vi "TLCCS Get Device Status.vi"(8 "error in (no error)":errorcluster {"code" format="%.0x"}, 11 "instrument handle":refnum<visa-resource-name>) -> (0 "error out":errorcluster {"code" format="%.0x"}, 2 "Device Status":i32, 3 "instrument handle out":refnum<visa-resource-name>)   [LabVIEW 2020]
doc: "This VI retrieves the status of the CCS. You can use this VI to detect if an external trigger has already occurred.\n\nNote:\nThe values anove are defined in the drivers header file."
uses:
  tlccs_32.dll
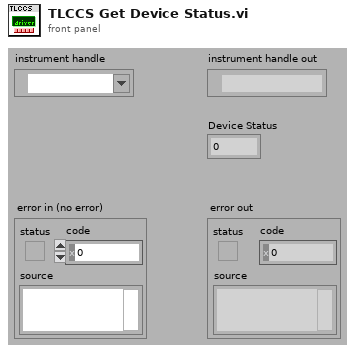
[diagram p1: front panel]
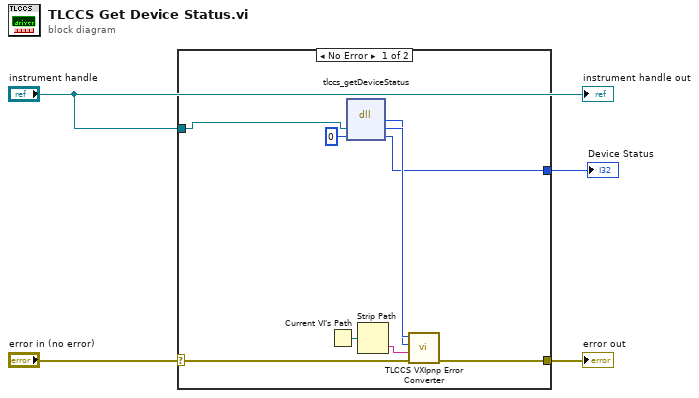
[diagram p0: block diagram]
diagram:
  n1 = case shown="No Error" "error in (no error)" {
    selector: "error in (no error)" -> [w8 w14]
    tunnel: [w7 w14] -> w4
    tunnel: "instrument handle" -> [w12 _]
    tunnel: [w5 _] -> w1
    frame No Error {
      n2 = Current VI's Path() -> (path=w13:path)
      n3 = dll-call lib="tlccs_32.*" fn="tlccs_getDeviceStatus"("Instrument Handle"=w12, "Device Status"=0) -> (w10:i32, "Instrument Handle"=w11:u32, "Device Status"=w5:i32)  [unwired: 3 in, 2 out]
      n4 = Strip Path(path=w13) -> (name=w9:string)  [unwired: 1 out]
      n5 = call "TLCCS VXIpnp Error Converter.vi"("error in (no error)"=w8, "name of VI (\"\")"=w9, "CVI error code (0)"=w10, "instrument handle"=w11) -> ("error out"=w7:errorcluster)  [unwired: 6 in, 1 out]
    }
    frame Error {
    }
  }
  "error out" <- w4
  "Device Status" <- w1
  "instrument handle out" <- "instrument handle"
